vi "Set speed.vi"(8 "error in (no error)":errorcluster, 11 "focus in":refnum<class "focus.lvclass">) -> (0 "error out":errorcluster, 3 "focus out":refnum<class "focus.lvclass">)   [LabVIEW 2012, in "focus.lvclass"]
uses:
  focus.lvclass
  focus.lvclass/focus.ctl
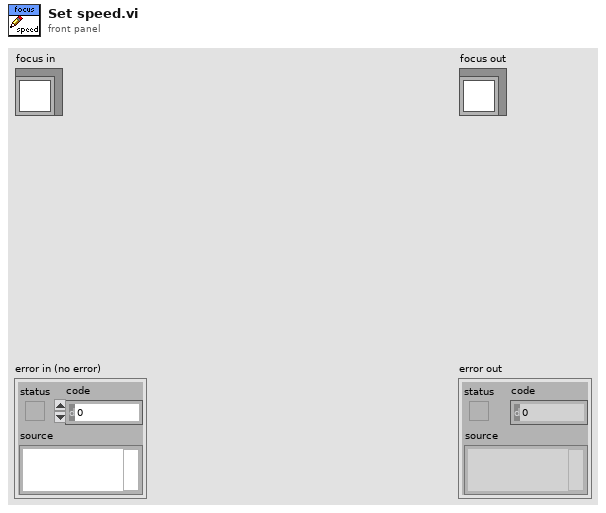
[diagram p1: front panel]
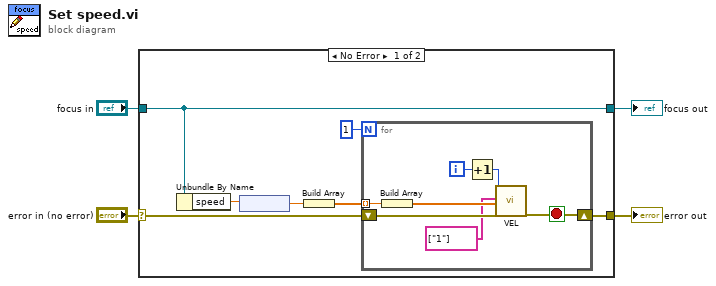
[diagram p0: block diagram]
diagram:
  n1 = case shown="No Error" "error in (no error)" {
    selector: "error in (no error)" -> [w6 w20]
    tunnel: [w5 w20] -> w3
    tunnel: [w11 w19] -> w1
    tunnel: "focus in" -> [w11 w19]
    frame No Error {
      n2 = Unbundle By Name(w11) -> ("speed"=w10:dbl[unit])
      n3 = node(w10) -> (w9:dbl)
      n4 = Build Array(w9) -> (w7:dbl[])
      n5 = for {
        N: 1 -> [_]
        tunnel: w7 -> [w18] mode=indexing
        shift-right: [w12] -> w5
        shift-left: w6 -> [w17]
        i -> [w14]
        stop <- w12 stop-if-true
        n6 = Build Array(w18) -> (w16:dbl[])
        n7 = Increment(x=w14) -> (x+1=w13:i32)
        n8 = call "VEL.vi"("System no."=w13, "Axes to set"=string[] ["1"], "Velocity values"=w16, "error in"=w17) -> ("error out"=w12:errorcluster)  [unwired: 14 in, 1 out]
      }
    }
    frame Error {
    }
  }
  "error out" <- w3
  "focus out" <- w1
